vi "ActionVIOnPaste_Good.vi"(6 "All Ptrs":T1[](array[typedef]) format="%.0x", 8 "error in (no error)":errorcluster, 10 "Parent":T1 format="%.0x", 11 "Ptr in":T1 format="%.0x") -> (0 "error out":errorcluster, 3 "Ptr out":T1 format="%.0x")   [LabVIEW 2027]
uses:
  <vilib>/NI VeriStand/Custom Device API/Custom Device Item Ref.ctl
  <vilib>/NI VeriStand/Custom Device API/Custom Device API.lvlib
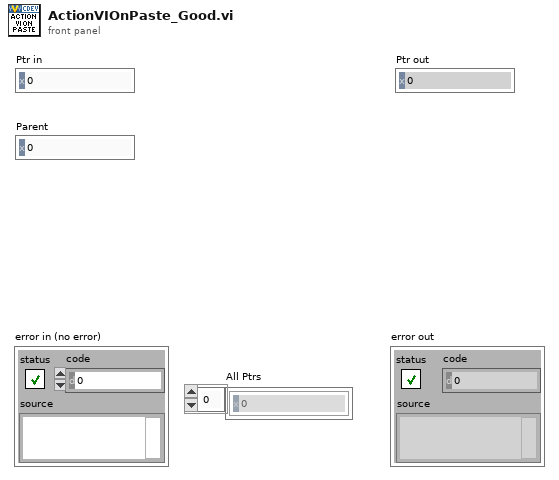
[diagram p1: front panel]
types:
  T1 = typedef "Custom Device API.lvlib/Custom Device Item Ref.ctl" = u64
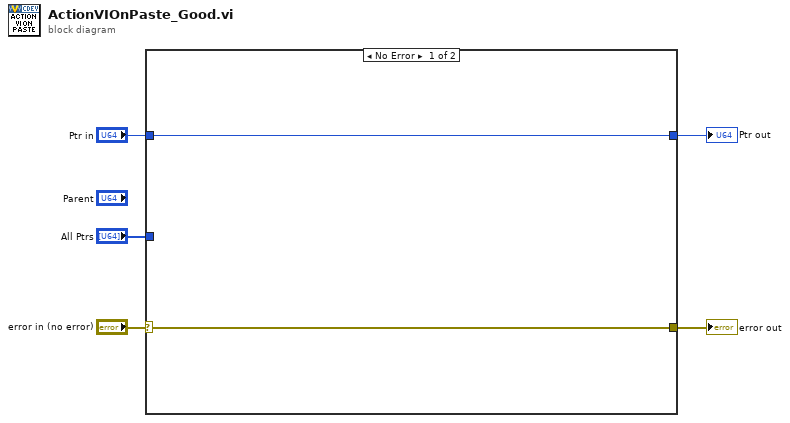
[diagram p0: block diagram]
diagram:
  n1 = case shown="No Error" "error in (no error)" {
    selector: "error in (no error)" -> [w7 w9]
    tunnel: [w7 w9] -> w4
    tunnel: "Ptr in" -> [w6 w8]
    tunnel: [w6 w8] -> w2
    tunnel: "All Ptrs" -> [_ _]
    frame No Error {
    }
    frame Error {
    }
  }
  "error out" <- w4
  "Ptr out" <- w2
